vi "MessbereichEinstellen_mitFrequenz.vi"(8 "Error_in":errorcluster, 10 "Channel Name (1: Channel 1)":i32(ring)=1 items=["Channel 1"=1, "Channel 2"=2, "Channel 3"=3, "Channel 4"=4], 11 "VISA Name OZ in(OZ)":refnum<visa-resource-name>="USB0::0x0957::0x179B::MY54313507::INSTR") -> (0 "Error_out":errorcluster, 3 "VISA Name OZ out":refnum<visa-resource-name>)   [LabVIEW 2016]
doc: "Mithilfe dieses VIs wird die Spannung des ausgewählten Channels auf 90% der Größe des Anzeigelements Skaliert."
panel:
  out "VPP":string
  out "Periodendauer [ms]":dbl
  out "Frequenz_alt":string
  out "Range_final":string
  out "RANGE 2":string
  out "Range_alt":string
  out "VMIN":string
  out "VMAX":string
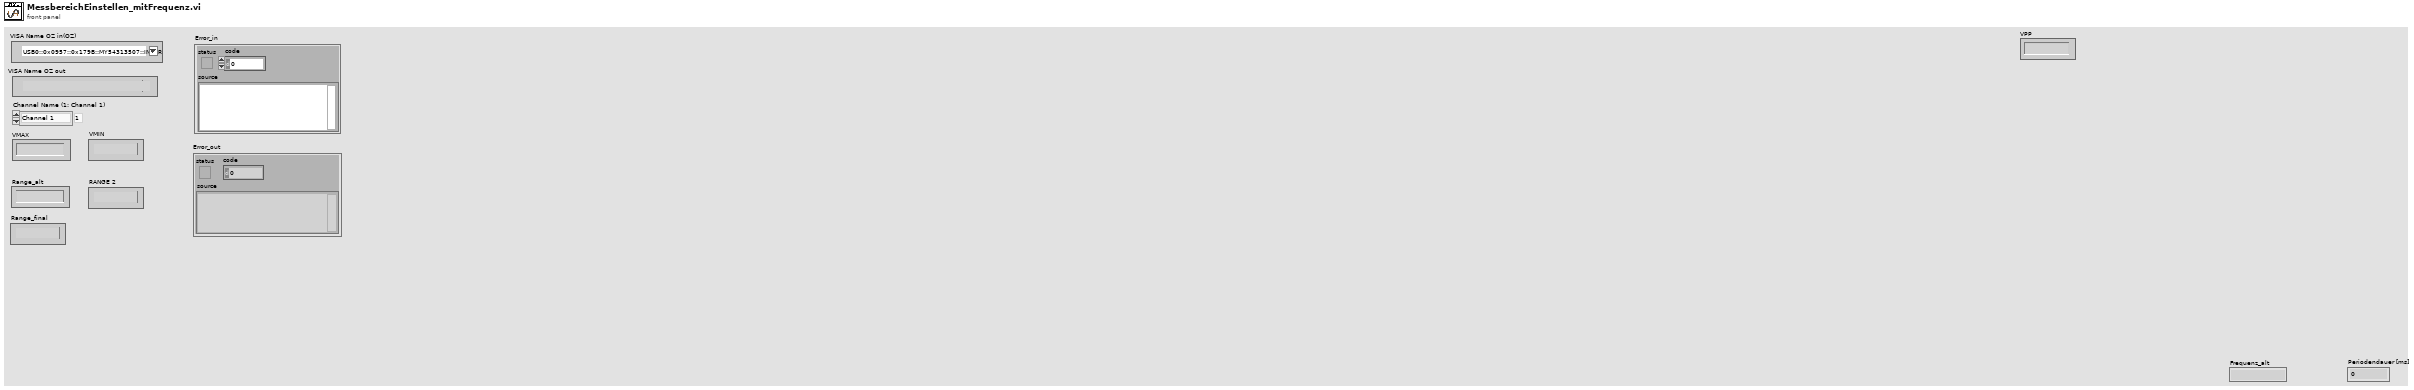
[diagram p1: front panel]
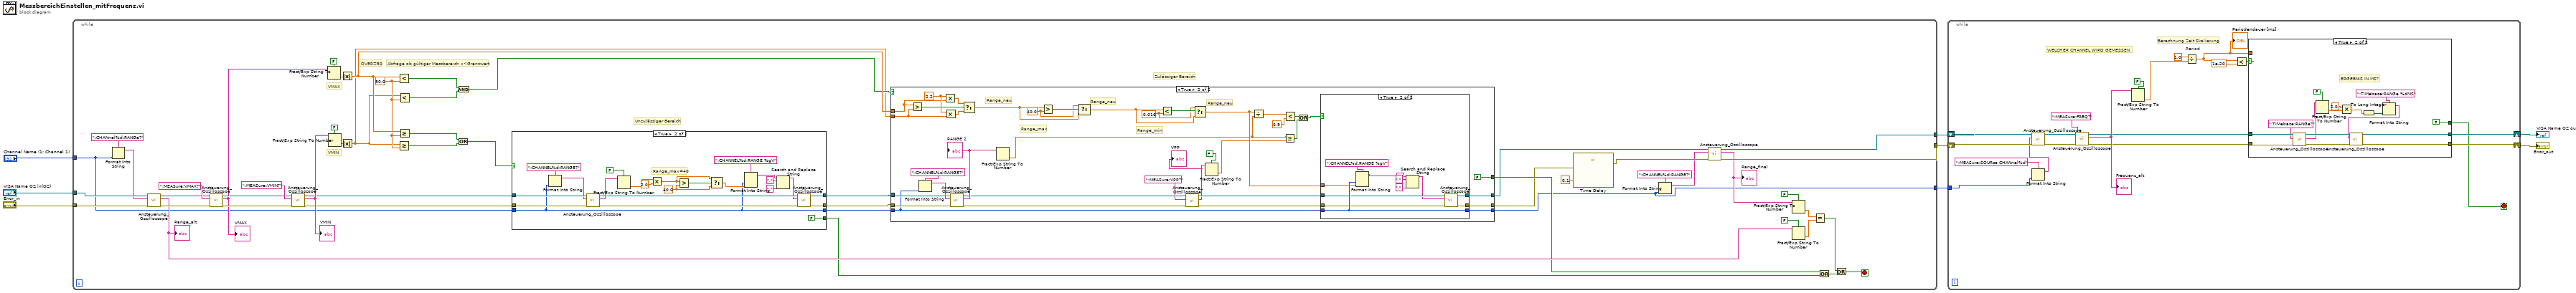
[diagram p0: block diagram]
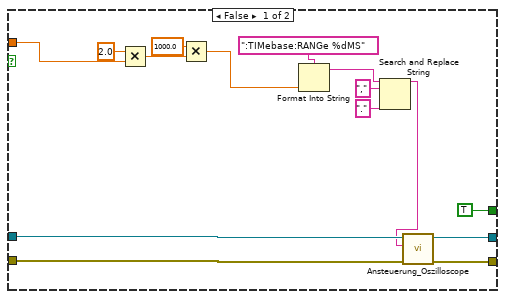
[diagram p2: hidden frame]
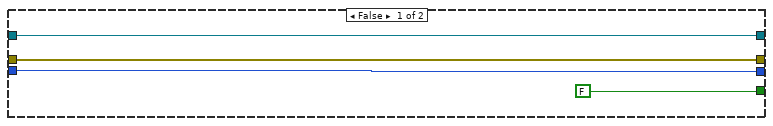
[diagram p3: hidden frame]
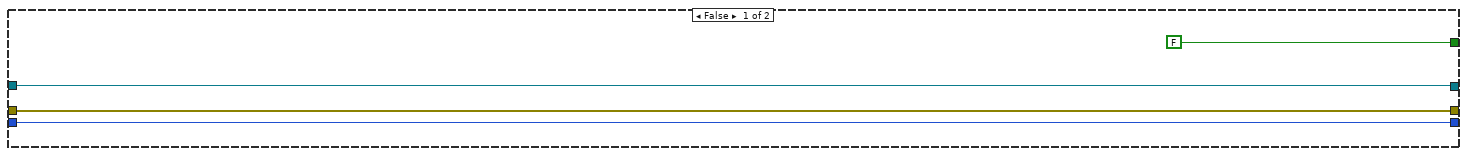
[diagram p4: hidden frame]
diagram:
  n1 = while {
    tunnel: "Error_in" -> [w43]
    tunnel: "VISA Name OZ in(OZ)" -> [w42]
    tunnel: "Channel Name (1: Channel 1)" -> [w15]
    tunnel: [w38] -> w5
    tunnel: [w36] -> w4
    tunnel: [w9] -> w1
    stop <- w25 stop-if-true
    w50 = 50.0 ("y")
    # "VMIN"
    # "VMAX"
    # "OVER=50"
    # "Unzulässiger Bereich"
    # "Zulässiger Bereich"
    # "Abfrage ob gültiger Messbereich x<Grenzwert"
    n2 = Format Into String(format string=":CHANnel%d:RANGe?" ("Schreibpuffer"), w15) -> (resulting string=w40:string)  [unwired: 2 in, 1 out]
    n3 = call "Ansteuerung_Oszilloscope.vi"("Error_in"=w43, "Eingangs-String"=w40, "VISA Name OZ in(OZ)"=w42) -> ("Error_out"=w44:errorcluster, "Ausgangs-String"=w31:string, "VISA Name OZ out"=w45:refnum<visa-resource-name>)  [unwired: 6 in]
    "Range_alt" <- w31
    n4 = call "Ansteuerung_Oszilloscope.vi"("Error_in"=w44, "Eingangs-String"=":MEASure:VMAX?" ("Schreibpuffer"), "VISA Name OZ in(OZ)"=w45) -> ("Error_out"=w59:errorcluster, "Ausgangs-String"=w55:string, "VISA Name OZ out"=w56:refnum<visa-resource-name>)  [unwired: 6 in]
    "VMAX" <- w55
    n5 = call "Ansteuerung_Oszilloscope.vi"("Error_in"=w59, "Eingangs-String"=":MEASure:VMIN?" ("Schreibpuffer"), "VISA Name OZ in(OZ)"=w56) -> ("Error_out"=w16:errorcluster, "Ausgangs-String"=w52:string, "VISA Name OZ out"=w17:refnum<visa-resource-name>)  [unwired: 6 in]
    "VMIN" <- w52
    n6 = Fract/Exp String To Number(use system decimal point (T)=FALSE, string=w55) -> (number=w23:dbl)  [unwired: 2 in, 1 out]
    n7 = Fract/Exp String To Number(use system decimal point (T)=FALSE, string=w52) -> (number=w22:dbl)  [unwired: 2 in, 1 out]
    n8 = Absolute Value(x=w23) -> (abs(x)=w51:dbl)
    n9 = Absolute Value(x=w22) -> (abs(x)=w10:dbl)
    n10 = Less?(x=w51, y=w50) -> (x < y?=w48:bool)
    n11 = Greater Or Equal?(x=w10, y=w50) -> (x >= y?=w46:bool)
    n12 = Less?(x=w10, y=w50) -> (x < y?=w49:bool)
    n13 = Greater Or Equal?(x=w51, y=w50) -> (x >= y?=w47:bool)
    n14 = Or(x=w47, y=w46) -> (x .or. y?=w14:bool)
    n15 = And(x=w48, y=w49) -> (x .and. y?=w21:bool)
    n16 = case shown="True" w14 {
      tunnel: w17 -> [w63 w86]
      tunnel: w16 -> [w62 w78]
      tunnel: w15 -> [w60 w68]
      tunnel: [FALSE FALSE] -> w11
      tunnel: [w62 w71] -> w19
      tunnel: [w63 w70] -> w20
      tunnel: [w60 w68] -> w18
      frame False {
      }
      frame True {
        w73 = 40.0 ("y")
        # "Range_max=40"
        n17 = Format Into String(format string=":CHANNEL%d:RANGE?" ("Schreibpuffer"), w68) -> (resulting string=w76:string)  [unwired: 2 in, 1 out]
        n18 = call "Ansteuerung_Oszilloscope.vi"("Error_in"=w78, "Eingangs-String"=w76, "VISA Name OZ in(OZ)"=w86) -> ("Error_out"=w79:errorcluster, "Ausgangs-String"=w84:string, "VISA Name OZ out"=w80:refnum<visa-resource-name>)  [unwired: 6 in]
        n19 = Fract/Exp String To Number(use system decimal point (T)=FALSE, string=w84) -> (number=w83:dbl)  [unwired: 2 in, 1 out]
        n20 = Multiply(x=w83, y=2.0) -> (x*y=w74:dbl)
        n21 = Greater?(x=w74, y=w73) -> (0:w75:bool)
        n22 = Select(t=w74, s=w75, f=w73) -> (s? t:f=w69:dbl)
        n23 = Format Into String(format string=":CHANNEL%d:RANGE %gV", w68, w69) -> (resulting string=w65:string)  [unwired: 2 in, 1 out]
        n24 = Search and Replace String(input string=w65, search string="," ("Such-String"), replace string="." ("Ersetzungs-String (\"\")")) -> (result string=w64:string)  [unwired: 5 in, 3 out]
        n25 = call "Ansteuerung_Oszilloscope.vi"("Error_in"=w79, "Eingangs-String"=w64, "VISA Name OZ in(OZ)"=w80) -> ("Error_out"=w71:errorcluster, "VISA Name OZ out"=w70:refnum<visa-resource-name>)  [unwired: 6 in, 1 out]
      }
    }
    n26 = case shown="True" w21 {
      tunnel: w20 -> [w90 w125]
      tunnel: [w90 w109] -> w13
      tunnel: w19 -> [w89 w124]
      tunnel: [w89 w108] -> w12
      tunnel: [w88 w107] -> w9
      tunnel: w18 -> [w88 w106]
      tunnel: [FALSE FALSE] -> w24
      tunnel: w10 -> [_ w117]
      tunnel: w23 -> [_ w116]
      frame False {
      }
      frame True {
        w111 = 0.016 ("y")
        w113 = 40.0 ("y")
        w118 = 2.2 ("y")
        # "Range_neu"
        # "Range_min"
        # "Range_neu"
        # "Range_max"
        # "Range_neu"
        n27 = Greater?(x=w116, y=w117) -> (0:w121:bool)
        n28 = Format Into String(format string=":CHANNEL%d:RANGE?" ("Schreibpuffer"), w106) -> (resulting string=w126:string)  [unwired: 2 in, 1 out]
        n29 = Multiply(x=w118, y=w116) -> (x*y=w120:dbl)
        n30 = Multiply(x=w118, y=w117) -> (x*y=w119:dbl)
        n31 = call "Ansteuerung_Oszilloscope.vi"("Error_in"=w124, "Eingangs-String"=w126, "VISA Name OZ in(OZ)"=w125) -> ("Error_out"=w97:errorcluster, "Ausgangs-String"=w123:string, "VISA Name OZ out"=w100:refnum<visa-resource-name>)  [unwired: 6 in]
        "RANGE 2" <- w123
        n32 = Select(t=w120, s=w121, f=w119) -> (s? t:f=w114:dbl)
        n33 = Fract/Exp String To Number(string=w123) -> (number=w95:dbl)  [unwired: 3 in, 1 out]
        n34 = Greater?(x=w114, y=w113) -> (0:w115:bool)
        n35 = Select(t=w113, s=w115, f=w114) -> (s? t:f=w110:dbl)
        n36 = Less?(x=w110, y=w111) -> (x < y?=w112:bool)
        n37 = call "Ansteuerung_Oszilloscope.vi"("Error_in"=w97, "Eingangs-String"=":MEASure:VPP?" ("Schreibpuffer"), "VISA Name OZ in(OZ)"=w100) -> ("Error_out"=w98:errorcluster, "Ausgangs-String"=w92:string, "VISA Name OZ out"=w99:refnum<visa-resource-name>)  [unwired: 6 in]
        "VPP" <- w92
        n38 = Select(t=w111, s=w112, f=w110) -> (s? t:f=w104:dbl)
        n39 = Fract/Exp String To Number(use system decimal point (T)=FALSE, string=w92) -> (number=w94:dbl)  [unwired: 2 in, 1 out]
        n40 = Divide(x=w104, y=w95) -> (x/y=w105:dbl)
        n41 = Less Or Equal?(x=w95, y=w94) -> (x <= y?=w93:bool)
        n42 = Less?(x=w105, y=0.9) -> (x < y?=w102:bool)
        n43 = Or(x=w102, y=w93) -> (x .or. y?=w103:bool)
        n44 = case shown="True" w103 {
          tunnel: [w130 w140] -> w109
          tunnel: [w129 w139] -> w108
          tunnel: [w128 w138] -> w107
          tunnel: w106 -> [w128 w138]
          tunnel: w99 -> [w130 w137]
          tunnel: w98 -> [w129 w136]
          tunnel: w104 -> [_ w135]
          frame False {
          }
          frame True {
            n45 = Format Into String(format string=":CHANNEL%d:RANGE %gV" ("Schreibpuffer"), w138, w135) -> (resulting string=w132:string)  [unwired: 2 in, 1 out]
            n46 = Search and Replace String(input string=w132, search string="," ("Such-String"), replace string="." ("Ersetzungs-String (\"\")")) -> (result string=w131:string)  [unwired: 5 in, 3 out]
            n47 = call "Ansteuerung_Oszilloscope.vi"("Error_in"=w136, "Eingangs-String"=w131, "VISA Name OZ in(OZ)"=w137) -> ("Error_out"=w139:errorcluster, "VISA Name OZ out"=w140:refnum<visa-resource-name>)  [unwired: 6 in, 1 out]
          }
        }
      }
    }
    n48 = call "Time Delay"("error in (no error)"=w12, "Delay Time (s)"=0.1) -> ("error out"=w37:errorcluster)  [unwired: 9 in]
    n49 = Format Into String(format string=":CHANNEL%d:RANGE?" ("Schreibpuffer"), w9) -> (resulting string=w34:string)  [unwired: 2 in, 1 out]
    n50 = call "Ansteuerung_Oszilloscope.vi"("Error_in"=w37, "Eingangs-String"=w34, "VISA Name OZ in(OZ)"=w13) -> ("Error_out"=w36:errorcluster, "Ausgangs-String"=w30:string, "VISA Name OZ out"=w38:refnum<visa-resource-name>)  [unwired: 6 in]
    "Range_final" <- w30
    n51 = Fract/Exp String To Number(use system decimal point (T)=FALSE, string=w30) -> (number=w29:dbl)  [unwired: 2 in, 1 out]
    n52 = Fract/Exp String To Number(use system decimal point (T)=FALSE, string=w31) -> (number=w28:dbl)  [unwired: 2 in, 1 out]
    n53 = Equal?(x=w29, y=w28) -> (x = y?=w26:bool)
    n54 = Or(x=w24, y=w11) -> (x .or. y?=w27:bool)
    n55 = Or(x=w26, y=w27) -> (x .or. y?=w25:bool)
  }
  n56 = while {
    shift-right: [w153] -> w2
    shift-left: w5 -> [w145]
    shift-right: [w154] -> w3
    shift-left: w4 -> [w146]
    tunnel: w1 -> [w142]
    stop <- w149 stop-if-true
    # "WELCHER CHANNEL WIRD GEMESSEN"
    # "Berechnung Zeit Skalierung"
    n57 = Format Into String(format string=":MEASure:SOURce CHANnel%d" ("Schreibpuffer"), w142) -> (resulting string=w143:string)  [unwired: 2 in, 1 out]
    n58 = call "Ansteuerung_Oszilloscope.vi"("Error_in"=w146, "Eingangs-String"=w143, "VISA Name OZ in(OZ)"=w145) -> ("Error_out"=w147:errorcluster, "VISA Name OZ out"=w148:refnum<visa-resource-name>)  [unwired: 6 in, 1 out]
    n59 = call "Ansteuerung_Oszilloscope.vi"("Error_in"=w147, "Eingangs-String"=":MEASure:FREQ?" ("Schreibpuffer"), "VISA Name OZ in(OZ)"=w148) -> ("Error_out"=w155:errorcluster, "Ausgangs-String"=w158:string, "VISA Name OZ out"=w156:refnum<visa-resource-name>)  [unwired: 6 in]
    "Frequenz_alt" <- w158
    n60 = Fract/Exp String To Number(use system decimal point (T)=FALSE ("Systemdezimalzeichen verwenden (T)"), string=w158) -> (number=w159:dbl)  [unwired: 2 in, 1 out]
    n61 = Divide "Period"(x=1.0, y=w159) -> (x/y=w151:dbl)
    "Periodendauer [ms]" <- w151
    n62 = Less?(x=w151, y=1e-20) -> (x < y?=w152:bool)
    n63 = case shown="True" w152 {
      tunnel: w151 -> [w168 _]
      tunnel: w156 -> [w167 w187]
      tunnel: w155 -> [w166 w188]
      tunnel: [w165 w189] -> w154
      tunnel: [w164 w190] -> w153
      tunnel: [TRUE FALSE] -> w149
      frame False {
        n64 = Multiply(x=2.0, y=w168) -> (x*y=w174:dbl)
        n65 = Multiply(x=1000.0, y=w174) -> (x*y=w173:dbl)
        n66 = Format Into String(format string=":TIMebase:RANGe %dMS" ("Schreibpuffer"), w173) -> (resulting string=w169:string)  [unwired: 2 in, 1 out]
        n67 = Search and Replace String(input string=w169, search string="," ("Such-String"), replace string="." ("Ersetzungs-String (\"\")")) -> (result string=w163:string)  [unwired: 5 in, 3 out]
        n68 = call "Ansteuerung_Oszilloscope.vi"("Error_in"=w166, "Eingangs-String"=w163, "VISA Name OZ in(OZ)"=w167) -> ("Error_out"=w165:errorcluster, "VISA Name OZ out"=w164:refnum<visa-resource-name>)  [unwired: 6 in, 1 out]
      }
      frame True {
        # "ERGEBNIS IN MS?"
        n69 = call "Ansteuerung_Oszilloscope.vi"("Error_in"=w188, "Eingangs-String"=":TIMebase:RANGe?" ("Schreibpuffer"), "VISA Name OZ in(OZ)"=w187) -> ("Error_out"=w191:errorcluster, "Ausgangs-String"=w184:string, "VISA Name OZ out"=w192:refnum<visa-resource-name>)  [unwired: 6 in]
        n70 = Fract/Exp String To Number(use system decimal point (T)=FALSE, string=w184) -> (number=w182:dbl)  [unwired: 2 in, 1 out]
        n71 = Multiply(x=2.0, y=w182) -> (x*y=w177:dbl)
        n72 = To Long Integer(number=w177) -> (32bit integer=w178:i32)
        n73 = Format Into String(format string=":TIMebase:RANGe %dMS" ("Schreibpuffer"), w178) -> (resulting string=w180:string)  [unwired: 2 in, 1 out]
        n74 = call "Ansteuerung_Oszilloscope.vi"("Error_in"=w191, "Eingangs-String"=w180, "VISA Name OZ in(OZ)"=w192) -> ("Error_out"=w189:errorcluster, "VISA Name OZ out"=w190:refnum<visa-resource-name>)  [unwired: 6 in, 1 out]
      }
    }
  }
  "VISA Name OZ out" <- w2
  "Error_out" <- w3
